vi "Generate String.vi"(8 "error in (no error)":errorcluster, 11 "object in":refnum<class "SetInputValue.lvclass">) -> (0 "error out":errorcluster, 2 "resulting string":string, 3 "object out":refnum<class "SetInputValue.lvclass">)   [LabVIEW 2017, in "SetInputValue.lvclass"]
uses:
  SetInputValue.lvclass
  SetInputValue.lvclass/SetInputValue.ctl
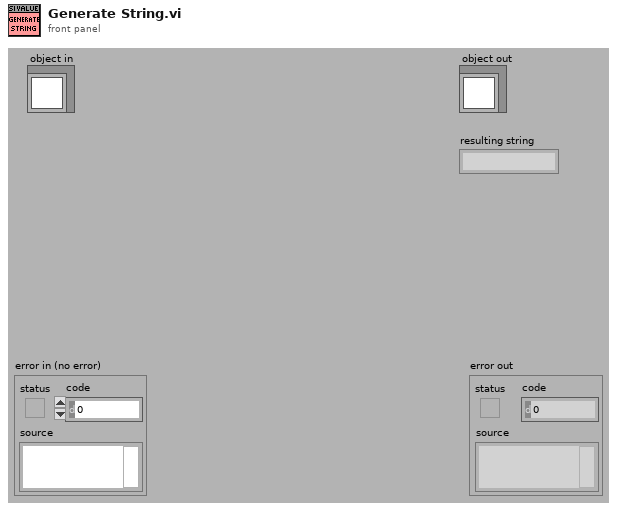
[diagram p1: front panel]
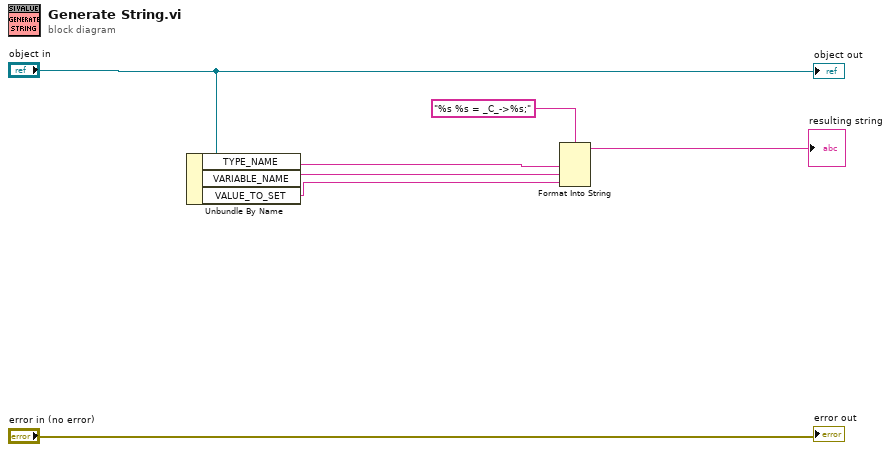
[diagram p0: block diagram]
diagram:
  n1 = Unbundle By Name("object in") -> ("TYPE_NAME"=w4:string, "VARIABLE_NAME"=w3:string, "VALUE_TO_SET"=w1:string)
  n2 = Format Into String(format string="%s %s = _C_->%s;", w4, w3, w1) -> (resulting string=→"resulting string":string)  [unwired: 2 in, 1 out]
  "error out" <- "error in (no error)"
  "object out" <- "object in"
